vi "1stAnd3rdorderFunc.vi"(0 "Y":dbl[](array[numeric]), 1 "X":dbl[](array[numeric]), 2 "Coefficients":dbl[](array[numeric])) -> (3 "Y converted":dbl[](array[numeric]), 4 "X converted":dbl[](array[numeric]), 5 "Residue":dbl[](array[numeric]), 6 "f(X,a)":dbl[](array[numeric]))   [LabVIEW 2020, in "XYcenter.lvlib"]
uses:
  XYcenter.lvlib
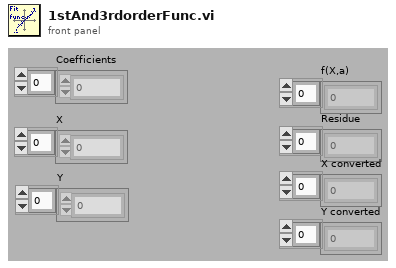
[diagram p1: front panel]
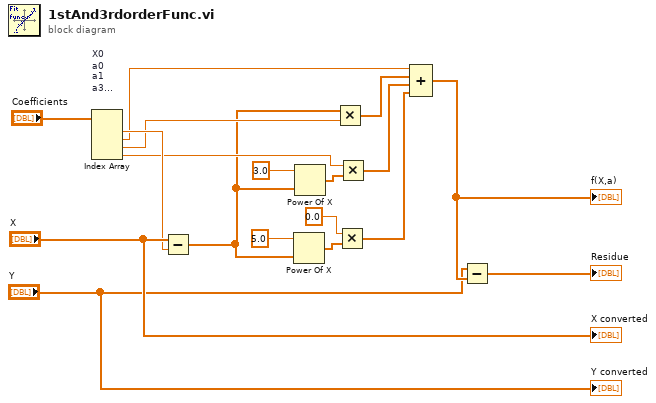
[diagram p0: block diagram]
diagram:
  n1 = Index Array "X0\na0\na1\na3\na5"(array="Coefficients") -> (element #1=w9:dbl, element #2=w8:dbl, element #3=w7:dbl, element #4=w6:dbl)  [unwired: 4 in]
  n2 = Subtract(x="X", y=w9) -> (x-y=w3:dbl[])
  n3 = Power Of X(1:w3, 2:5.0) -> (0:w4:dbl[])
  n4 = Power Of X(1:w3, 2:3.0) -> (0:w16:dbl[])
  n5 = Multiply(x=w3, y=w7) -> (x*y=w15:dbl[])
  n6 = Multiply(x=0.0, y=w4) -> (x*y=w2:dbl[])
  n7 = Multiply(x=w6, y=w16) -> (x*y=w14:dbl[])
  n8 = Compound Arithmetic op=ADD(w8, w15, w14, w2) -> (w13:dbl[])
  "f(X,a)" <- w13
  n9 = Subtract(x="Y", y=w13) -> (x-y=→"Residue":dbl[])
  "X converted" <- "X"
  "Y converted" <- "Y"
